vi "OpenLabViewIniWithCode.vi"   [LabVIEW 2020]
uses:
  846b9cc9-b277-4677-9e2a-d5b282abfd94.vi
  <resource>/dialog/lvconfig.llb/LV Config Read String.vi
types:
  T1 = enum32{"Invalid", "Standard", "Closed", "Hidden", "Minimized", "Maximized"}
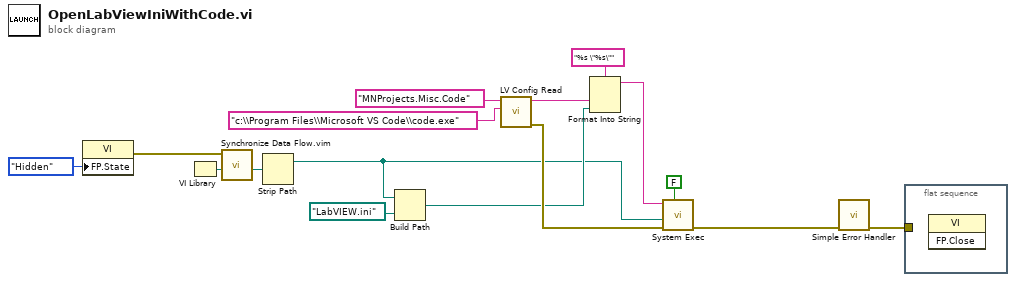
[diagram p0: block diagram]
diagram:
  n1 = property class="VI"("FP.State"=T1."Hidden" ("Front Panel Window:State")) -> (error out=w1:errorcluster)  [unwired: 2 in, 1 out]
  n2 = VI Library() -> (path=w7:path)
  n3 = call "Synchronize Data Flow.vim"("input 3"=w7, "input 1"=w1) -> ("output 3"=w3:path)  [unwired: 2 in, 3 out]
  n4 = Strip Path(path=w3) -> (stripped path=w4:path)  [unwired: 1 out]
  n5 = Build Path(base path=w4, name or relative path=path "LabVIEW.ini") -> (appended path=w5:path)
  n6 = call-poly <resource>:"LV Config Read.vi"("default value"="c:\\Program Files\\Microsoft VS Code\\code.exe" ("command line"), "key"="MNProjects.Misc.Code") -> ("error out"=w12:errorcluster, "value"=w9:string)  [unwired: 3 in, 1 out]
  n7 = Format Into String(format string="%s \"%s\"", w9, w5) -> (resulting string=w8:string)  [unwired: 2 in, 1 out]
  n8 = call <vilib>:"System Exec.vi"("wait until completion? (T)"=FALSE, "error in (no error)"=w12, "working directory"=w4, "command line"=w8) -> ("error out"=w15:errorcluster)  [unwired: 4 in, 3 out]
  n9 = call <vilib>:"Simple Error Handler.vi"("error in (no error)"=w15) -> ("error out"=w11:errorcluster)  [unwired: 4 in, 4 out]
  n10 = flat-sequence {
    tunnel: w11 -> [_]
    frame #0 {
      n11 = invoke class="VI" method="FP.Close"() -> ()  [unwired: 3 in, 3 out]
    }
  }
